vi "Konvolucio MUDS150628 B232EATC Read DTC.vi"() -> ()   [LabVIEW 2011]
uses:
  <instrlib>/Konvolucio MUDS150628/Konvolucio MUDS150628.lvlib
panel:
  out "Response":string
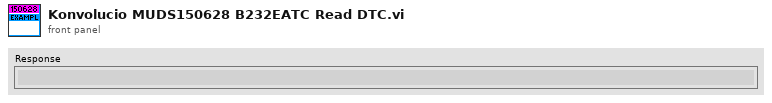
[diagram p1: front panel]
types:
  T1 = typedef "Konvolucio MUDS150628.lvlib/UdsHandleType.ctl" = cluster{"LogPath":path, "LogEnabled":bool, "isOpen":bool, "LogContent":string, "Adapter":string, "MCanHandle":T2, "TransmittId":u32, "ReceiveId":u32}
  T2 = typedef "Konvolucio MCAN120803.lvlib/MCanHandleType.ctl" = cluster{"MCanAdapter":refnum<k24>}
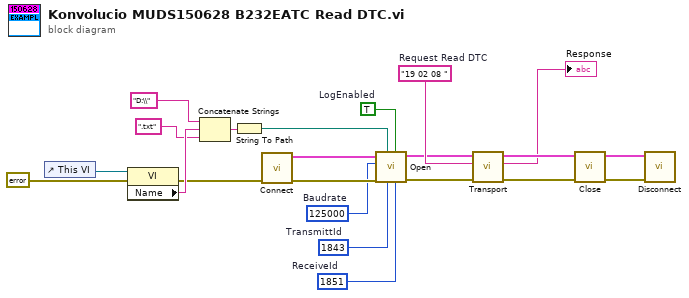
[diagram p0: block diagram]
diagram:
  w10 = TRUE  # LogEnabled
  w9 = u32 125000  # Baudrate
  w6 = u32 1851  # ReceiveId
  w7 = u32 1843  # TransmittId
  w19 = "19 02 08 "  # Request Read DTC
  n1 = control-ref of="This VI"() -> (w18:refnum<vi>)
  n2 = property class="VI"(reference=w18, error in=errorcluster {"status"=FALSE, "code"=0, "source"=""} ("error in (no error)")) -> (error out=w13:errorcluster, "Name"=w16:string)  [unwired: 1 out]
  n3 = Concatenate Strings("D:\\" ("VI Name"), w16, ".txt" ("string")) -> (w14:string)
  n4 = String To Path(string=w14) -> (path=w8:path)
  n5 = call <instrlib>:"Connect.vi"("error in"=w13) -> ("error out"=w11:errorcluster, "UdsHandleOut"=w12:T1)  [unwired: 9 in]
  n6 = call <instrlib>:"Open.vi"("ReceiveId"=w6, "LogEnabled"=w10, "TransmittId"=w7, "LogPath"=w8, "error in"=w11, "BaudRate"=w9, "UdsHandleIn"=w12) -> ("error out"=w4:errorcluster, "UdsHandleOut"=w3:T1)  [unwired: 3 in]
  n7 = call <instrlib>:"Transport.vi"("error in"=w4, "Request"=w19, "UdsHandleIn"=w3) -> ("error out"=w22:errorcluster, "Response"=→"Response":string, "UdsHandleOut"=w21:T1)  [unwired: 6 in]
  n8 = call <instrlib>:"Close.vi"("error in"=w22, "UdsHandleIn"=w21) -> ("error out"=w2:errorcluster, "UdsHandleOut"=w1:T1)  [unwired: 8 in]
  n9 = call <instrlib>:"Disconnect.vi"("error in"=w2, "UdsHandleIn"=w1) -> ()  [unwired: 9 in, 1 out]
